vi "Create Or Replace File.vi"(8 "error in (no error)":errorcluster, 10 "logfilename.txt":path, 11 "relative file path":path) -> (0 "error out":errorcluster, 3 "Byte Stream File out":refnum<file>)   [LabVIEW 2020, in "RxnRover.lvlib" / "File IO.lvlib"]
doc: "Creates a file of specified name at type at a relative location appended with the aboslute Local App State Data Path\n\nCreated 5/20/2025 - Labview 2020\nRxnRover"
uses:
  File IO.lvlib
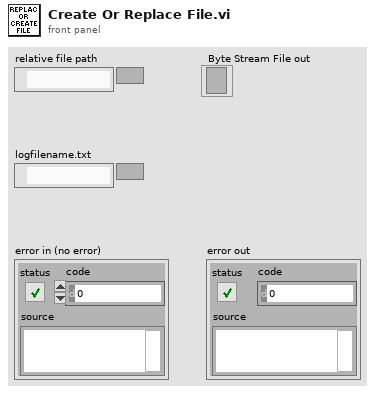
[diagram p1: front panel]
types:
  T1 = enum16{"open", "replace", "create", "open or create", "replace or create", "replace or create with confirmation"}
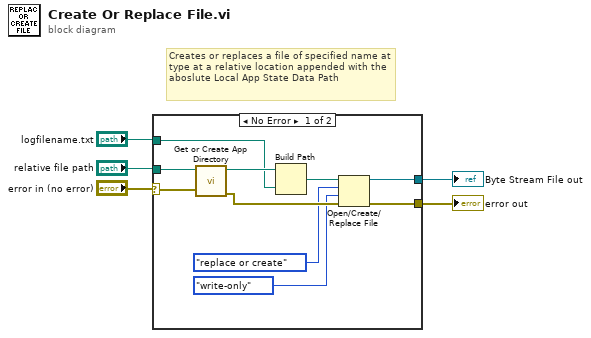
[diagram p0: block diagram]
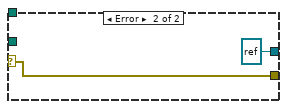
[diagram p2: hidden frame]
diagram:
  # "Creates or replaces a file of specified name at type at a relative location appended with the aboslute Local App State Data Path"
  n1 = case shown="No Error" "error in (no error)" {
    selector: "error in (no error)" -> [w9 w17]
    tunnel: "logfilename.txt" -> [w10 _]
    tunnel: "relative file path" -> [w8 _]
    tunnel: [w7 w17] -> w2
    tunnel: [w6 refnum<file> refnum ("refnum out")] -> w1
    frame No Error {
      n2 = call "Get or Create App Directory.vi"("error in (no error)"=w9, "Relative Path"=w8) -> ("error out"=w15:errorcluster, "Ouput File Path"=w11:path)  [unwired: 8 in]
      n3 = Build Path(base path=w11, name or relative path=w10) -> (appended path=w12:path)
      n4 = Open/Create/Replace File(file path (use dialog)=w12, error in=w15, operation (0:open)=T1."replace or create", access (0:read/write)=enum16{"read/write", "read-only", "write-only"}."write-only") -> (refnum out=w6:refnum<file>, error out=w7:errorcluster)  [unwired: 2 in, 1 out]
    }
    frame Error {
    }
  }
  "Byte Stream File out" <- w1
  "error out" <- w2
